vi "fpga_96ch-Super_mux_sched.vi"(1 "12 8Ch-timestamp-data array":T1[](array[typedef])=[{"Timestamp"=0, "Data available"=FALSE}, {"Timestamp"=0, "Data available"=FALSE}, {"Timestamp"=0, "Data available"=FALSE}, {"Timestamp"=0, "Data available"=FALSE}, {"Timestamp"=0, "Data available"=FALSE}, {"Timestamp"=0, "Data available"=FALSE}, {"Timestamp"=0, "Data available"=FALSE}, {"Timestamp"=0, "Data available"=FALSE}, {"Timestamp"=0, "Data available"=FALSE}, {"Timestamp"=0, "Data available"=FALSE}, {"Timestamp"=0, "Data available"=FALSE}, {"Timestamp"=0, "Data available"=FALSE}], 2 "Scheduler":u8) -> (0 "All Ch Timestamps":T1={"Timestamp"=0, "Data available"=TRUE})   [LabVIEW 2011]
uses:
  lib/Time Stamp Data.ctl
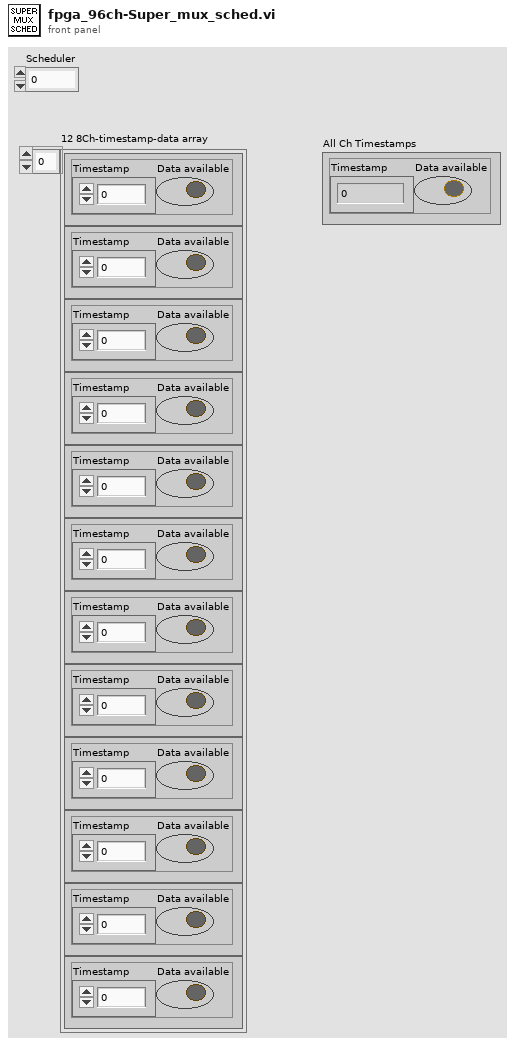
[diagram p1: front panel]
types:
  T1 = typedef "Time Stamp Data.ctl" = cluster{"Timestamp":u32, "Data available":bool}
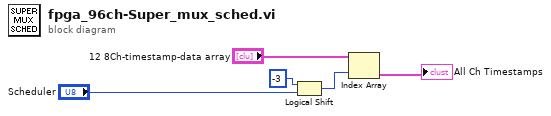
[diagram p0: block diagram]
diagram:
  n1 = Logical Shift(y=i8 -3, x="Scheduler") -> (x << y=w1:u8)
  n2 = Index Array(array="12 8Ch-timestamp-data array", index=w1) -> (element=→"All Ch Timestamps":T1)
